vi "Configure DAQmx DCPower Synchronization.vi"(0 "DCPower Trigger Destination":T1, 1 "Connect?":bool, 5 "DAQ Trigger Source":T6, 11 "error in (no error)":errorcluster) -> (15 "error out":errorcluster)   [LabVIEW 2020]
uses:
  Common/Instrument Control/DAQmx/Pin Map/TSM DAQmx Multi-Task.ctl
  <vilib>/NI_TestStand_SemiconductorModule/NI_TestStand_Semiconductor_Module.lvlibp/PinMap/PinQueryContext/MultiplePinMultipleSessionQueryContext/MultiplePinMultipleSessionQueryContext.lvclass
  Common/Instrument Control/DAQmx/Pin Map/SSC DAQmx.ctl
  Common/Instrument Control/DCPower/TSM/TSM SSC DCPower.ctl
  Common/Instrument Control/DCPower/SSC DCPower/SSC DCPower.ctl
  Common/Instrument Control/Shared SubVIs/TSM Pin Abstraction/TSM Pin Information.ctl
  Common/Instrument Control/Shared SubVIs/TSM Pin Abstraction/TSM Pin Type Identifier.ctl
  Common/Instrument Control/Shared SubVIs/TSM Pin Abstraction/TSM Expanded Pin Information.ctl
  <instrlib>/niDCPower/nidcpower.llb/niDCPower Configure Digital Edge Source Trigger With Channels.vi
  <instrlib>/niDCPower/nidcpower.llb/niDCPower Disable Source Trigger With Channels.vi
  <resource>/objmgr/daqmx.rc
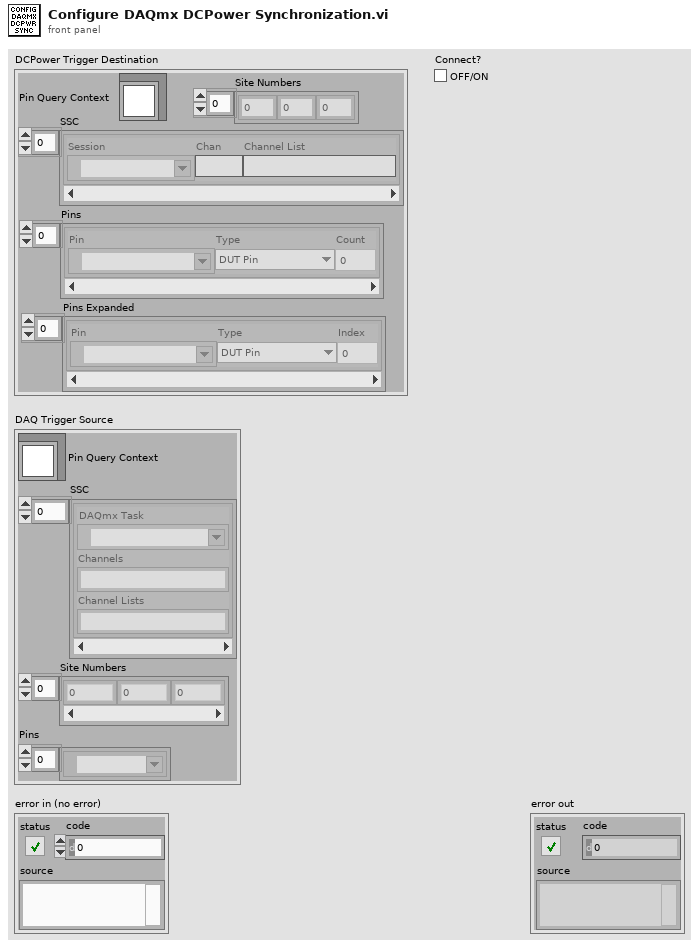
[diagram p1: front panel]
types:
  T1 = typedef "TSM SSC DCPower.ctl" = cluster{"Pin Query Context":refnum<class "MultiplePinMultipleSessionQueryContext.lvclass">, "SSC":T2[], "Site Numbers":i32[], "Pins":T3[], "Pins Expanded":T5[]}
  T2 = typedef "SSC DCPower.ctl" = cluster{"Session":refnum<k15>, "Chan":string, "Channel List":string}
  T3 = typedef "TSM Pin Information.ctl" = cluster{"Pin":tag, "Type":T4, "Count":i32}
  T4 = typedef "TSM Pin Type Identifier.ctl" = enum8{"DUT Pin", "System Pin", "Pin Group", "Not Determined"}
  T5 = typedef "TSM Expanded Pin Information.ctl" = cluster{"Pin":tag, "Type":T4, "Index":i32}
  T6 = typedef "TSM DAQmx Multi-Task.ctl" = cluster{"Pin Query Context":refnum<class "MultiplePinMultipleSessionQueryContext.lvclass">, "SSC":T7[], "Site Numbers":i32[], "Pins":tag[]}
  T7 = typedef "SSC DAQmx.ctl" = cluster{"DAQmx Task ":refnum<k21>, "Channels":string, "Channel Lists":string}
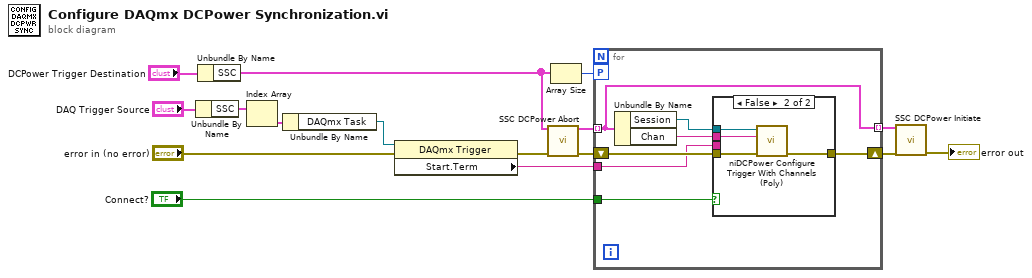
[diagram p0: block diagram]
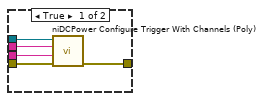
[diagram p2: hidden frame]
diagram:
  n1 = Unbundle By Name("DAQ Trigger Source") -> ("SSC"=w14:T7[])
  n2 = Unbundle By Name("DCPower Trigger Destination") -> ("SSC"=w7:T2[])
  n3 = Index Array(array=w14) -> (element=w13:T7)  [unwired: 1 in]
  n4 = Unbundle By Name(w13) -> ("DAQmx Task"=w12:refnum<k21>)
  n5 = property class="DAQmx Trigger"(reference=w12, error in="error in (no error)") -> (error out=w10:errorcluster, "Start.Term"=w5:tag)  [unwired: 1 out]
  n6 = call "SSC DCPower Abort.vi"("DCPower SSC in"=w7, "error in"=w10) -> ("DCPower SSC out"=w8:T2[], "error out"=w9:errorcluster)  [unwired: 12 in]
  n7 = Array Size(array=w7) -> (size(s)=w6:i32)
  n8 = for {
    tunnel: w8 -> [w18] mode=indexing
    workers-P: w6 -> [_]
    tunnel: w5 -> [w20]
    shift-right: [w19] -> w4
    shift-left: w9 -> [w23]
    tunnel: [w18] -> w3 mode=indexing
    tunnel: "Connect?" -> [w17]
    n9 = Unbundle By Name(w18) -> ("Session"=w22:refnum<k15>, "Chan"=w21:string)
    n10 = case shown="False" w17 {
      tunnel: w23 -> [w28 w32]
      tunnel: w22 -> [w27 w31]
      tunnel: w21 -> [w26 w30]
      tunnel: w20 -> [w25 _]
      tunnel: [w24 w29] -> w19
      frame True {
        n11 = call-poly <instrlib>:"niDCPower Configure Trigger With Channels (Poly).vi"("error in (no error)"=w28, "input terminal"=w25, "channel name"=w26, "instrument handle"=w27) -> ("error out"=w24:errorcluster)  [unwired: 6 in, 1 out]
      }
      frame False {
        n12 = call-poly <instrlib>:"niDCPower Configure Trigger With Channels (Poly).vi"("error in (no error)"=w32, "channel name"=w30, "instrument handle"=w31) -> ("error out"=w29:errorcluster)  [unwired: 7 in, 1 out]
      }
    }
  }
  n13 = call "SSC DCPower Initiate.vi"("DCPower SSC in"=w3, "error in"=w4) -> ("error out"=→"error out":errorcluster)  [unwired: 12 in, 1 out]
